vi "Prompt for Step New.vi"(8 "error in (no error)":errorcluster, 9 "Index":i32=-1, 11 "Steps":refnum<class "Step.lvclass">[](array[class])) -> (0 "error out":errorcluster, 1 "OK?":bool, 3 "Step":refnum<class "Step.lvclass">)   [LabVIEW 2020, in "MacroAssert.lvlib"]
doc: "Prompts to enter a new step in the profile."
uses:
  MacroAssert.lvlib
  Classes/Step/Step.lvclass
  CTLs/Step Type V3.ctl
  CTLs/Assertion Type.ctl
  CTLs/Prompt for Step State Data.ctl
  FaKI State Machine/FaKI State Machine.lvlib
  CTLs/Prompt for Step Front Panel Data.ctl
  <vilib>/Utility/inputDevices.llb/mouseAcquire.vi
  <vilib>/Utility/inputDevices.llb/closeMouse.vi
  <vilib>/picture/picture.llb/imagedata.ctl
  Classes/Macro/Macro.lvclass
  CTLs/Step V3.ctl
panel:
  in  "Save Default":bool
  in  "Step Notes":string
  out "Step Type Description":string
  in  "Repeat Amount":i32 min=0
  in  "Tab Control":T1(tab)
  in  "Y":i32 min=0
  in  "X":i32 min=0
  in  "Right Click?":bool
  in  "Key":u8(ring)=65
  in  "App/Window Name":string
  in  "Stop on Fail?":bool
  in  "Control Name":string
  in  "Tab Control 2":T2(tab)
  in  "Disabled":T3(ring)
  in  "Visible":enum16{"Visible", "Not Visible"}(ring)
  in  "Left":i16
  in  "Top":i16
  in  "Width":i16
  in  "Height":i16
  out "Expected Image":picture
  in  "Delay (ms)":i32=100 min=0
  in  "Step Type":T4
  in  "Cancel":bool
  in  "OK":bool caption="OK2"
  # "Left and right click at\nsame time to capture\ncurrent screen coords"
  # "Left and right click at\nsame time to capture\nexpected value"
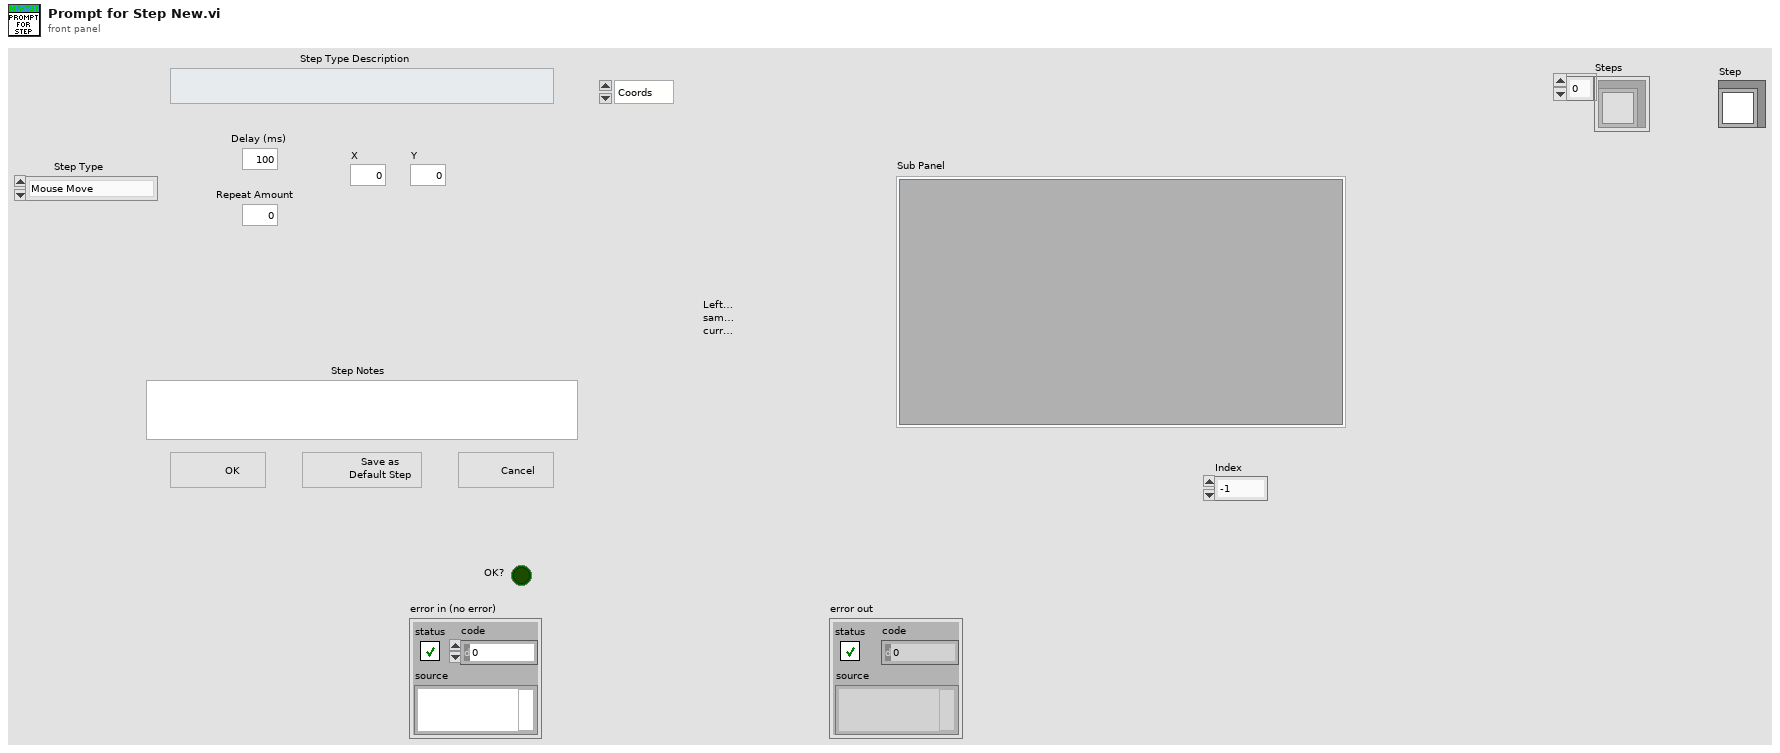
[diagram p1: front panel]
types:
  T1 = enum32{"Coords", "RClick", "Key", "A/W", "Nothing", "Assertion"}
  T2 = enum32{"Control Position", "Control Disabled", "Control Visible", "Control Image"}
  T3 = enum8{"Enabled", "Disabled", "Disabled and Grayed Out"}
  T4 = typedef "MacroAssert.lvlib/Step Type V3.ctl" = enum16{"Mouse Move", "Mouse Click", "Key Press", "Wait", "Mouse Down", "Mouse Up", "Key Down", "Key Up", "Maximize Window", "Restore Window", "Minimize Window", "Close Window", "Bring Window to Front", "Send Window to Back", "Assertion: Ctl Visible", "Assertion: Ctl Disabled", "Assertion: Ctl Image"}
  T5 = typedef "MacroAssert.lvlib/Prompt for Step State Data.ctl" = cluster{"Core":cluster{"Current VI Reference":refnum<vi>, "Close Panel on Exit?":bool}, "Mouse Ref":refnum<k1>, "Step":refnum<class "Step.lvclass">, "FP":T6, "OK?":bool}
  T6 = typedef "MacroAssert.lvlib/Prompt for Step Front Panel Data.ctl" = cluster{"Assertion Type":T7, "Step":T8}
  T7 = typedef "MacroAssert.lvlib/Assertion Type.ctl" = enum16{"Control Position", "Control Visible", "Control Disabled", "Control Image"}
  T8 = typedef "MacroAssert.lvlib/Step V3.ctl" = cluster{"Type":T4, "X":i32, "Y":i32, "Delay":i32, "Key":u8, "Repeat":i32, "RClick?":bool, "App/Window Name":string, "Notes":string, "Assertion Type":T7, "Control Name":string, "Stop on Fail?":bool, "Disabled":enum8{"Enabled", "Disabled", "Disabled and Grayed Out"}, "Visible":enum16{"Visible", "Not Visible"}, "Left":i16, "Top":i16, "Width":i16, "Height":i16, "Expected Image":T9}
  T9 = typedef "imagedata.ctl" = cluster{"image type":i32, "image depth":i32, "image":u8[], "mask":u8[], "colors":u32[], "Rectangle":cluster{"left":i16, "top":i16, "right":i16, "bottom":i16}}
  T10 = enum32{"Invalid", "Standard", "Closed", "Hidden", "Minimized", "Maximized"}
  T11 = enum32{"invalid app kind", "Development System", "Run Time System", "Student Edition", "Embedded LabVIEW", "Evaluation", "Custom"}
  T12 = enum32{"Coords", "RClick", "Key", "A/W", "Nothing"}
  T13 = cluster{"Horizontal":i32, "Vertical":i32, "Scrolling":i32}
  T14 = cluster{"button 1":bool, "button 2":bool, "button 3":bool, "button 4":bool}
  T15 = cluster{"left":i16, "top":i16, "right":i16, "bottom":i16}
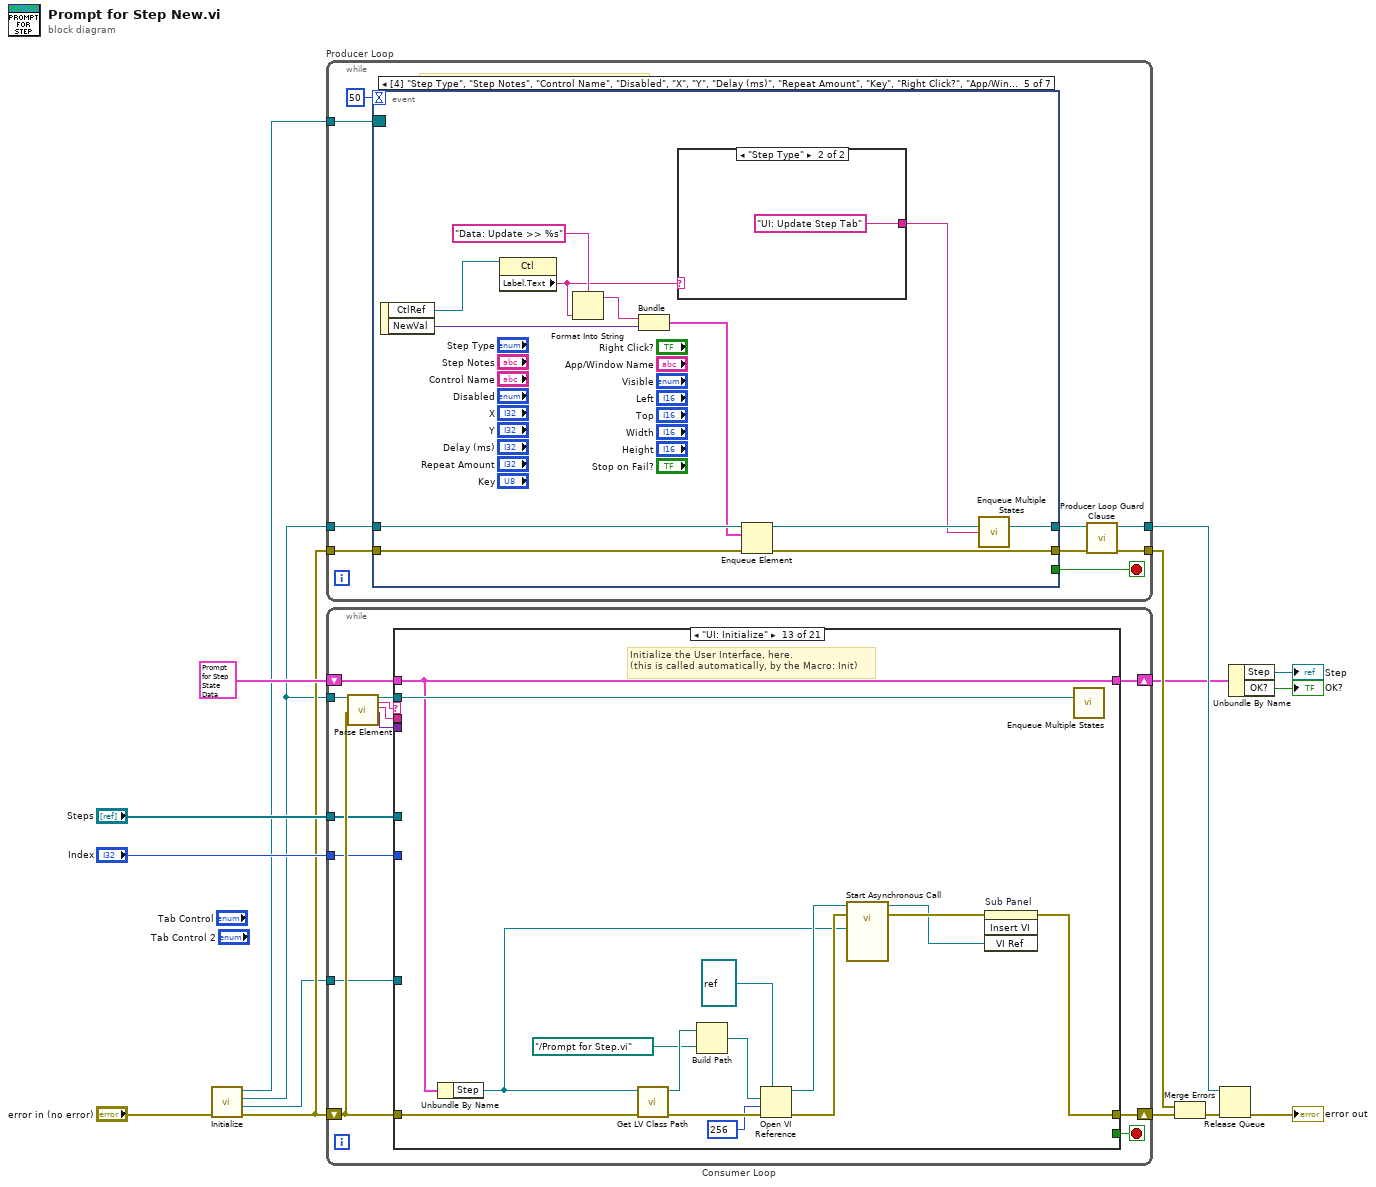
[diagram p0: block diagram]
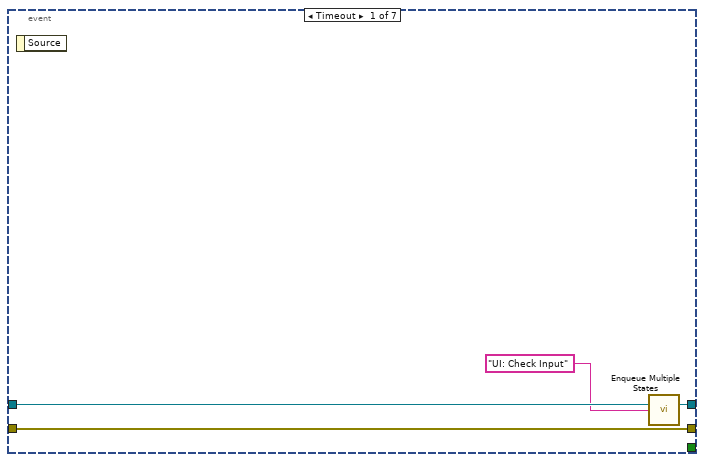
[diagram p2: hidden frame]
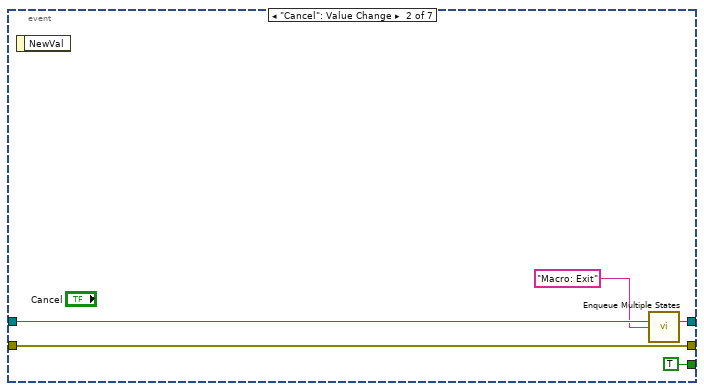
[diagram p3: hidden frame]
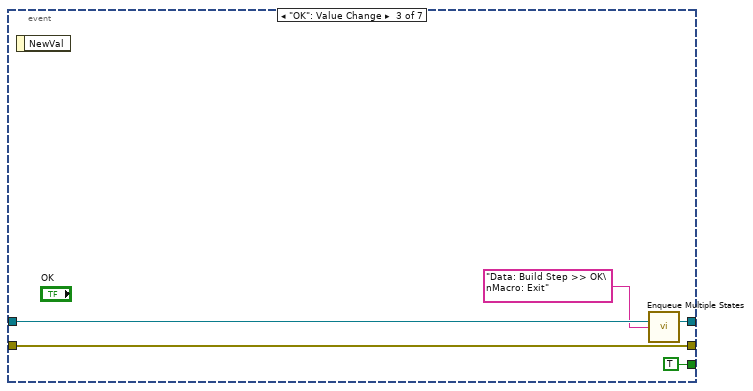
[diagram p4: hidden frame]
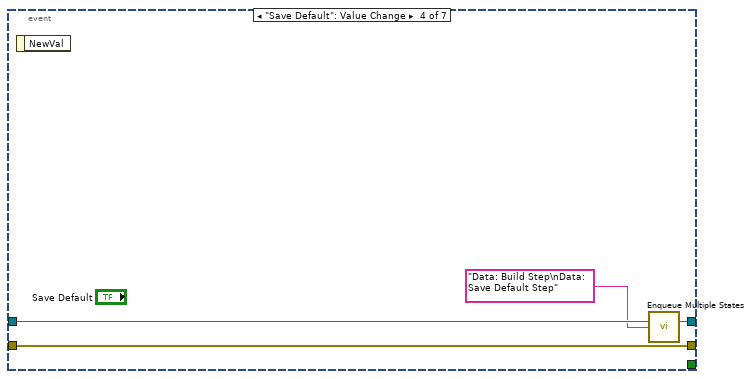
[diagram p5: hidden frame]
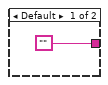
[diagram p6: hidden frame]
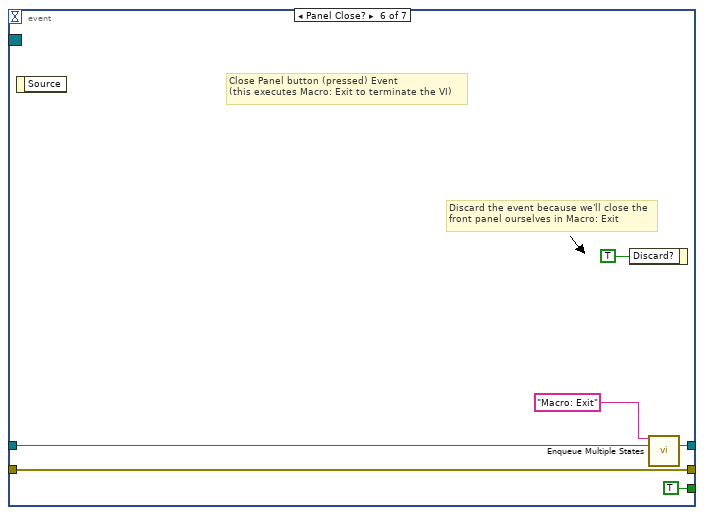
[diagram p7: hidden frame]
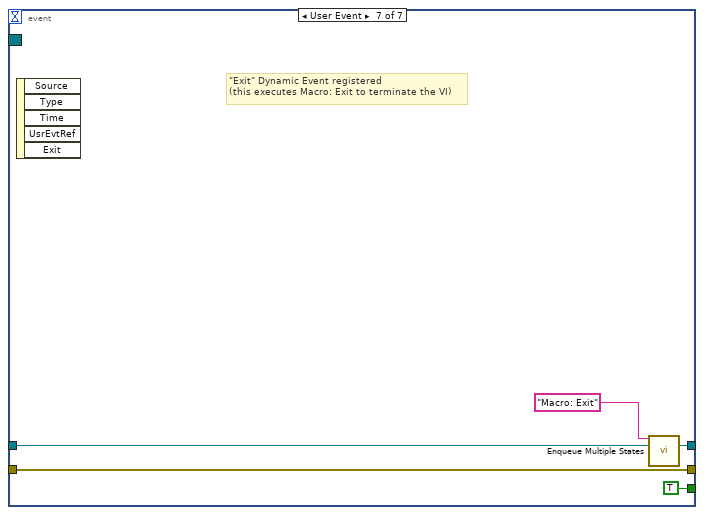
[diagram p8: hidden frame]
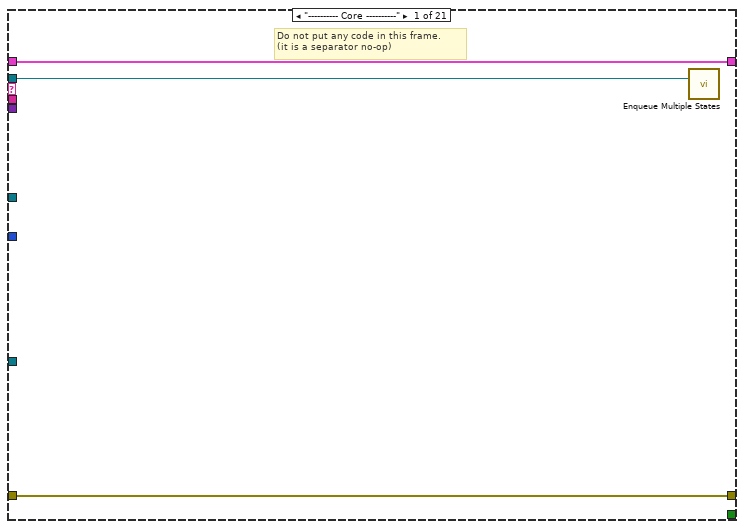
[diagram p9: hidden frame]
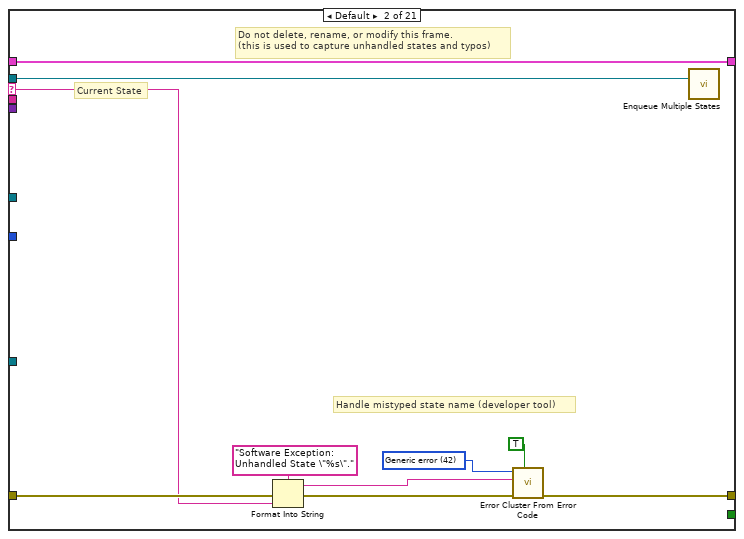
[diagram p10: hidden frame]
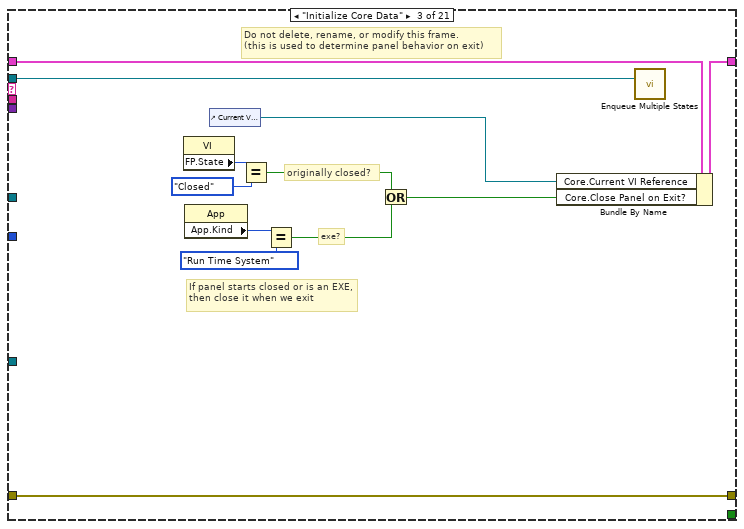
[diagram p11: hidden frame]
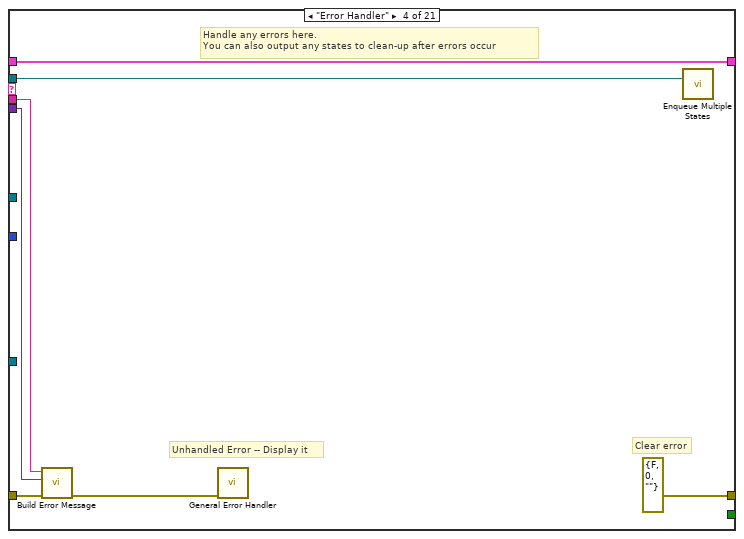
[diagram p12: hidden frame]
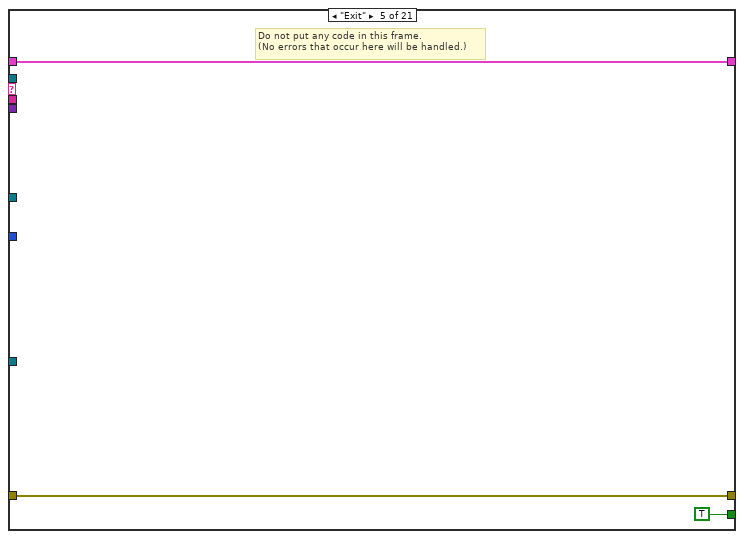
[diagram p13: hidden frame]
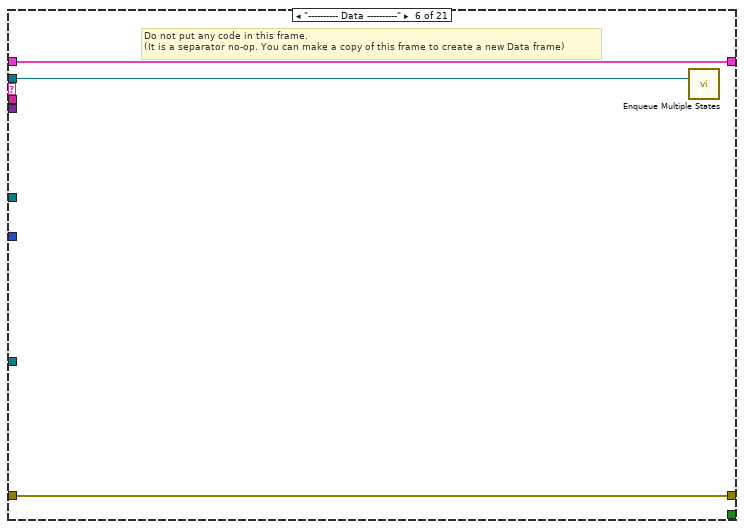
[diagram p14: hidden frame]
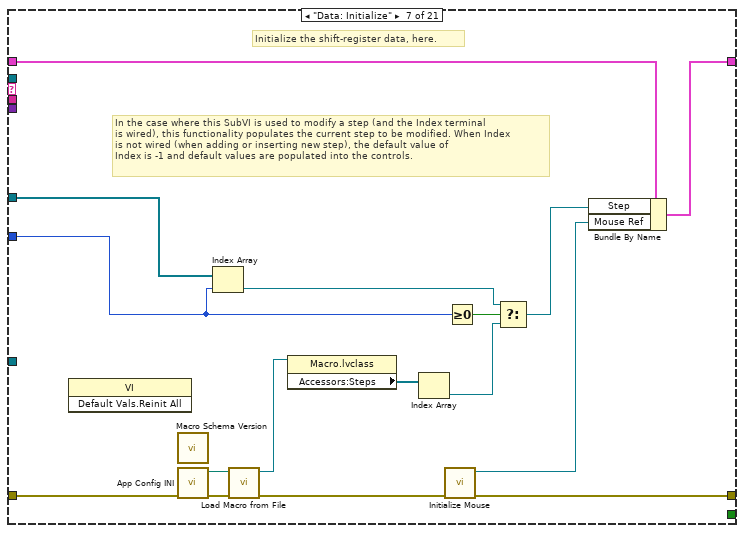
[diagram p15: hidden frame]
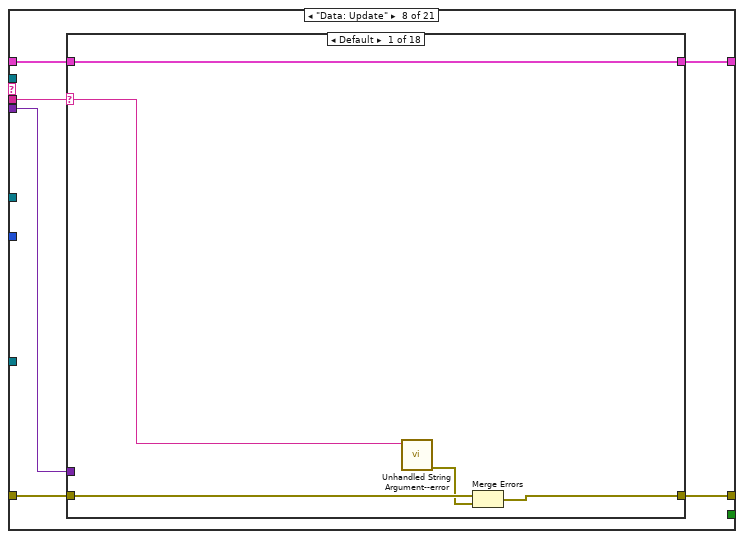
[diagram p16: hidden frame]
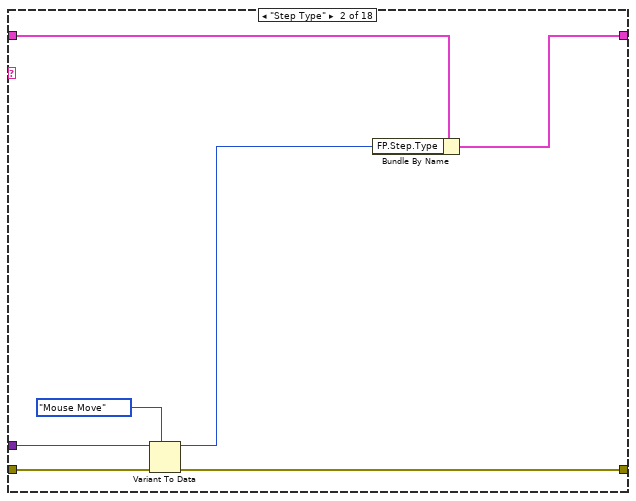
[diagram p17: hidden frame]
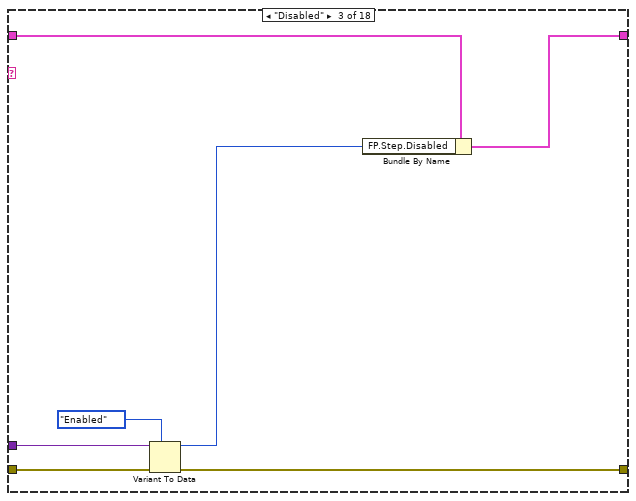
[diagram p18: hidden frame]
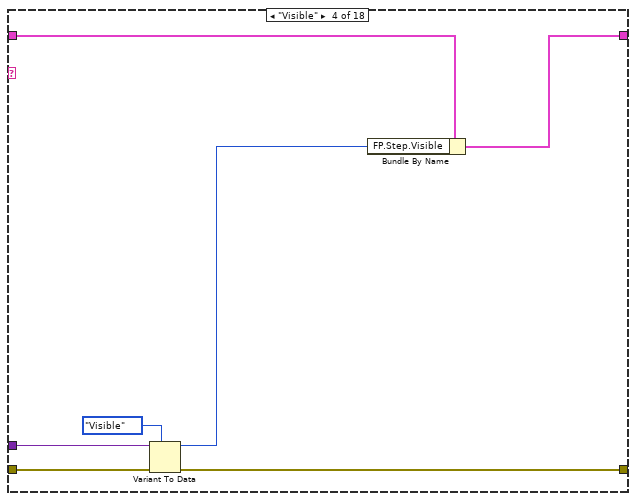
[diagram p19: hidden frame]
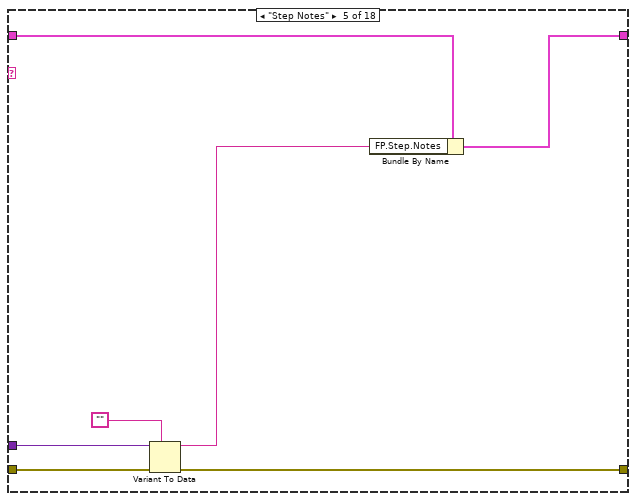
[diagram p20: hidden frame]
diagram:
  n1 = call "Initialize.vi"("error in (no error)"="error in (no error)") -> ("error out"=w5:errorcluster, "Exit Event"=w4:refnum<user-event>, "Queue"=w3:refnum<queue>, "Event Registration Refnum"=w2:refnum<event-registration>)  [unwired: 7 in]
  n2 = while "Producer Loop" {
    tunnel: w2 -> [w17]
    tunnel: w3 -> [w21]
    tunnel: [w18] -> w12
    tunnel: w5 -> [w25]
    tunnel: [w23] -> w15
    stop <- w20 stop-if-true
    # "executes when the state queue is empty"
    n3 = event shown="[4] \"Step Type\", \"Step Notes\", \"Control Name\", \"Disabled\", \"X\", \"Y\", \"Delay (ms)\", \"Repeat Amount\", \"Key\", \"Right Click?\", \"App/Window Name\", \"Visible\", \"Left\", \"Top\", \"Width\", \"Height\", \"Stop on Fail?\": Value Change" {
      selector: w17 -> [_ _ _ _ _ _ _]
      dyn-events: _ -> [_ _ _ _ _ _ _]
      timeout: 50 ("Timeout") -> [_ _ _ _ _ _ _]
      tunnel: [w29 w34 w39 w43 w54 w63 w68] -> w24
      tunnel: w25 -> [w29 w34 w39 w43 w55 w63 w68]
      tunnel: w21 -> [w27 w33 w38 w42 w53 w60 w66]
      tunnel: [w28 w32 w37 w41 w44 w59 w65] -> w19
      tunnel: [_ TRUE TRUE _ _ TRUE TRUE] -> w20
      event Timeout {
        n4 = event-data() -> ()  [unwired: 1 in, 1 out]
        n5 = call "Enqueue Multiple States.vi"("queue in"=w27, "State(s) at Back"="UI: Check Input") -> ("queue out"=w28:refnum<queue>)  [unwired: 13 in]
      }
      event "Cancel": Value Change {
        n6 = event-data() -> ()  [unwired: 1 in, 1 out]
        n7 = call "Enqueue Multiple States.vi"("queue in"=w33, "State(s) at Back"="Macro: Exit") -> ("queue out"=w32:refnum<queue>)  [unwired: 13 in]
      }
      event "OK": Value Change {
        n8 = event-data() -> ()  [unwired: 1 in, 1 out]
        n9 = call "Enqueue Multiple States.vi"("queue in"=w38, "State(s) at Back"="Data: Build Step >> OK\nMacro: Exit") -> ("queue out"=w37:refnum<queue>)  [unwired: 13 in]
      }
      event "Save Default": Value Change {
        n10 = event-data() -> ()  [unwired: 1 in, 1 out]
        n11 = call "Enqueue Multiple States.vi"("queue in"=w42, "State(s) at Back"="Data: Build Step\nData: Save Default Step") -> ("queue out"=w41:refnum<queue>)  [unwired: 13 in]
      }
      event "Step Notes", "Control Name", "Disabled", "X", "Y", "Delay (ms)", "Repeat Amount", "Key", "Right Click?", "App/Window Name", "Visible", "Left", "Top", "Width", "Height", "Stop on Fail?": Value Change {
        n12 = event-data() -> ("CtlRef"=w45:refnum<vi>, "NewVal"=w46:variant)  [unwired: 1 in]
        n13 = property class="Ctl"(reference=w45) -> ("Label.Text"=w48:string)  [unwired: 1 in, 2 out]
        n14 = Format Into String(format string="Data: Update >> %s", w48) -> (resulting string=w49:string)  [unwired: 2 in, 1 out]
        n15 = Bundle(w49, "NewVal"=w46) -> (w47:cluster{string, "NewVal":variant})  [unwired: 1 in]
        n16 = case shown="\"Step Type\"" w48 {
          tunnel: ["" ("string") "UI: Update Step Tab" ("string")] -> w51
          frame Default {
          }
          frame "Step Type" {
          }
        }
        n17 = Enqueue Element(queue=w53, element=w47, error in (no error)=w55) -> (queue out=w52:refnum<queue>, error out=w54:errorcluster)  [unwired: 1 in, 1 out]
        n18 = call "Enqueue Multiple States.vi"("queue in"=w52, "State(s) at Back"=w51) -> ("queue out"=w44:refnum<queue>)  [unwired: 13 in]
      }
      event Panel Close? {
        # "Discard the event because we'll close the front panel ourselves in Macro: Exit"
        # "Close Panel button (pressed) Event\n(this executes Macro: Exit to terminate the VI)"
        n19 = event-data() -> ()  [unwired: 1 in, 1 out]
        n20 = event-data("Discard?"=TRUE) -> ()  [unwired: 1 in, 1 out]
        n21 = call "Enqueue Multiple States.vi"("State(s) at Front"="Macro: Exit", "queue in"=w60) -> ("queue out"=w59:refnum<queue>)  [unwired: 13 in]
      }
      event User Event {
        # "\"Exit\" Dynamic Event registered\n(this executes Macro: Exit to terminate the VI)"
        n22 = event-data() -> ()  [unwired: 1 in, 5 out]
        n23 = call "Enqueue Multiple States.vi"("State(s) at Front"="Macro: Exit", "queue in"=w66) -> ("queue out"=w65:refnum<queue>)  [unwired: 13 in]
      }
    }
    n24 = call "Producer Loop Guard Clause.vi"("error in (no error)"=w24, "queue in"=w19) -> ("error out"=w23:errorcluster, "queue out"=w18:refnum<queue>)  [unwired: 8 in]
  }
  n25 = while "Consumer Loop" {
    shift-right: [w78] -> w8
    shift-left: T5 {"Core"={"Current VI Reference"=refnum, "Close Panel on Exit?"=FALSE}, "Mouse Ref"=refnum, "Step"=refnum, "FP"={"Assertion Type"=enum."Control Position", "Step"={"Type"=enum."Mouse Move", "X"=0, "Y"=0, "Delay"=0, "Key"=0, "Repeat"=0, "RClick?"=FALSE, "App/Window Name"="", "Notes"="", "Assertion Type"=enum."Control Position", "Control Name"="", "Stop on Fail?"=FALSE, "Disabled"=enum."Enabled", "Visible"=enum."Visible", "Left"=0, "Top"=0, "Width"=0, "Height"=0, "Expected Image"={"image type"=0, "image depth"=0, "image"=[], "mask"=[], "colors"=[], "Rectangle"={"left"=0, "top"=0, "right"=0, "bottom"=0}}}}, "OK?"=FALSE} ("Prompt for Step State Data") -> [w69]
    shift-right: [w81] -> w16
    shift-left: w5 -> [w80]
    tunnel: w3 -> [w77]
    tunnel: w4 -> [w72]
    tunnel: "Steps" -> [w71]
    tunnel: "Index" -> [w70]
    stop <- w79 stop-if-true
    n26 = call "Parse Element.vi"("queue in"=w77, "error in (no error)"=w80) -> ("queue out"=w76:refnum<queue>, "State"=w75:string, "Arg"=w74:string, "Data"=w73:variant)  [unwired: 14 in]
    n27 = case shown="\"UI: Initialize\"" w75 {
      selector: w75 -> [_ w86 _ _ _ _ _ _ _ _ _ _ _ _ _ _ _ _ _ _ _]
      tunnel: w76 -> [w82 w85 w95 w109 _ w117 _ _ _ _ w291 w297 w314 w317 w318 w327 _ _ w496 w501 w507]
      tunnel: w74 -> [_ _ _ w107 _ _ _ w138 _ w285 _ _ _ _ w319 w328 _ _ _ _ _]
      tunnel: w69 -> [w83 w88 w101 w110 w115 w118 w133 w139 w275 w287 w292 w298 w308 w316 w320 w330 w400 w443 w497 w500 w511]
      tunnel: [w84 w93 w106 errorcluster {"status"=FALSE, "code"=0, "source"=""} ("error out") w116 w119 w134 w140 w268 w279 w294 w299 w300 w315 w321 w331 w403 w445 w498 w502 w512] -> w81
      tunnel: w80 -> [w84 w92 w106 w112 w116 w119 w135 w141 w276 w282 w296 w299 w309 w315 w322 w332 w403 w446 w498 w502 w512]
      tunnel: [_ _ _ _ TRUE _ _ _ _ _ _ _ _ _ _ _ _ _ _ _ _] -> w79
      tunnel: [w83 w88 w105 w110 w115 w118 w132 w136 w275 w286 w292 w298 w308 w316 w320 w330 w400 w442 w497 w500 w511] -> w78
      tunnel: w73 -> [_ _ _ w108 _ _ _ w137 _ _ _ _ _ _ _ _ _ _ _ _ _]
      tunnel: w72 -> [_ _ _ _ _ _ _ _ _ _ _ _ _ _ _ _ _ _ _ _ _]
      tunnel: w71 -> [_ _ _ _ _ _ w129 _ _ _ _ _ _ _ _ _ _ _ _ _ _]
      tunnel: w70 -> [_ _ _ _ _ _ w128 _ _ _ _ _ _ _ _ _ _ _ _ _ _]
      frame "---------- Core ----------" {
        # "Do not put any code in this frame.\n(it is a separator no-op)"
        n28 = call "Enqueue Multiple States.vi"("queue in"=w82) -> ()  [unwired: 14 in, 1 out]
      }
      frame Default {
        w90 = 42 items=["No error", "Argument error", "Memory is full", "Out of zone", "End of file", "File already open", "Generic file I/O error", "File not found", "File permission error", "Disk is full", "Duplicate path", "Too many files open", "System feature not enabled", "Resource file not found", "Cannot add resource", "Resource not found", "Image not found", "Image memory error", "Pen does not exist", "Config type invalid", "Config token not found", "Config parse error", "Config memory error", "Bad external code format", "Bad external code offset", "External code not present", "Null window", "Destroy window error", "Null menu", "Print aborted", "Bad print record", "Print driver error", "Windows error during printing", "Memory error during printing", "Print dialog error", "Generic print error", "Invalid device refnum", "Device not found", "Device parameter error", "Device unit error", "Cannot open device", "Device call aborted", "Generic error", "Cancelled by user", "Object ID too low", "Object ID too high", "Object not in heap", "Unknown heap", "Unknown object (invalid DefProc)", "Unknown object (DefProc not in table)", "Message out of range", "Invalid (null) method", "Unknown message", "Manager call not supported", "Bad address", "Network operation in progress", "Network operation timed out", "Connection is busy", "Network attribute not supported", "Network error", "Address in use", "System out of memory", "Connection aborted", "Connection refused", "Not connected", "Already connected", "Connection closed", "Initialization error (interapplication manager)", "Bad occurrence", "Wait on unbound occurrence handler", "Occurrence queue overflow", "Datalog type conflict", "Unused", "Unrecognized type (interapplication manager)", "Memory corrupt", "Failed to make temporary DLL", "Old CIN version", "Drag socket not found", "Failed to load drop-object", "Failed to register OLE object", "Failed to release OLE object", "Format specifier type mismatch", "Unknown format specifier", "Too few format specifiers", "Too many format specifiers", "Scan failed", "Newer CIN version", "Error converting to variant", "Runtime menu error", "Password tampered", "Variant attribute not found", "Incompatible variant data type", "Event data is not available", "Event Store is not present", "Occurrence is not found", "Event Queue is not created", "Event info is not available", "Refnum passed is NULL", "Error retrieving Class GUID", "Error retrieving CoClass GUID", "Error retrieving TypeLib GUID.", "Bad built application magic bytes.", "Specific driver is different from the specific driver associated with the Logical Name.", "There is no session opened to the class driver.", "Max Error", "MAX - Error with config objects", "MAX - Error loading configuration", "MAX - Group not supported"]
        # "Current State"
        # "Do not delete, rename, or modify this frame.\n(this is used to capture unhandled states and typos)"
        # "Handle mistyped state name (developer tool)"
        n29 = Format Into String(format string="Software Exception: Unhandled State \"%s\"." ("message"), error in=w92, w86) -> (resulting string=w89:string, error out=w94:errorcluster)  [unwired: 1 in]
        n30 = call <vilib>:"Error Cluster From Error Code.vi"("show call chain? (False)"=TRUE, "error in (no error)"=w94, "error message (\"\")"=w89, "error code (0)"=w90) -> ("error out"=w93:errorcluster)  [unwired: 5 in]
        n31 = call "Enqueue Multiple States.vi"("queue in"=w85) -> ()  [unwired: 14 in, 1 out]
      }
      frame "Initialize Core Data" {
        # "Do not delete, rename, or modify this frame.\n(this is used to determine panel behavior on exit)"
        # "originally closed?"
        # "exe?"
        # "If panel starts closed or is an EXE, then close it when we exit"
        n32 = property class="VI"() -> ("FP.State"=w98:T10)  [unwired: 2 in, 2 out]
        n33 = property class="App"() -> ("App.Kind"=w104:T11)  [unwired: 2 in, 2 out]
        n34 = control-ref of="Current VI Reference"() -> (w99:refnum<vi>)
        n35 = Equal?(x=w98, y=T10."Closed" ("Front Panel Window:State")) -> (x = y?=w96:bool)
        n36 = Equal?(x=w104, y=T11."Run Time System" ("Application:Kind")) -> (x = y?=w102:bool)
        n37 = Or(x=w96, y=w102) -> (x .or. y?=w100:bool)
        n38 = Bundle By Name(cluster=w101, "Core.Current VI Reference"=w99, "Core.Close Panel on Exit?"=w100) -> (w105:T5)
        n39 = call "Enqueue Multiple States.vi"("queue in"=w95) -> ()  [unwired: 14 in, 1 out]
      }
      frame "Error Handler" {
        # "Unhandled Error -- Display it"
        # "Handle any errors here.\nYou can also output any states to clean-up after errors occur"
        # "Clear error"
        n40 = call "Build Error Message.vi"("error in (no error)"=w112, "Data"=w108, "Arg"=w107) -> ("error out"=w111:errorcluster)  [unwired: 8 in]
        n41 = call <vilib>:"General Error Handler.vi"("error in (no error)"=w111) -> ()  [unwired: 10 in, 5 out]
        n42 = call "Enqueue Multiple States.vi"("queue in"=w109) -> ()  [unwired: 14 in, 1 out]
      }
      frame "Exit" {
        # "Do not put any code in this frame.\n(No errors that occur here will be handled.)"
      }
      frame "---------- Data ----------" {
        # "Do not put any code in this frame.\n(It is a separator no-op. You can make a copy of this frame to create a new Data frame)"
        n43 = call "Enqueue Multiple States.vi"("queue in"=w117) -> ()  [unwired: 14 in, 1 out]
      }
      frame "Data: Initialize" {
        # "In the case where this SubVI is used to modify a step (and the Index terminal\nis wired), this functionality populates the current step to be modified. When Index\nis not wired (when adding or inserting new step), the default value of\nIndex is -1 and default values are populated into the controls."
        # "Initialize the shift-register data, here."
        n44 = invoke class="VI" method="Default Vals.Reinit All"() -> ()  [unwired: 3 in, 3 out]
        n45 = call "Macro Schema Version.vi"() -> ()  [unwired: 10 in, 2 out]
        n46 = call "App Config INI.vi"("error in (no error)"=w135) -> ("error out"=w125:errorcluster, "App Config"=w124:path)  [unwired: 9 in]
        n47 = Index Array(array=w129, index=w128) -> (element=w131:refnum<class "Step.lvclass">)
        n48 = call "Load Macro from File.vi"("error in (no error)"=w125, "Path"=w124) -> ("error out"=w123:errorcluster, "Macro"=w121:refnum<class "Macro.lvclass">)  [unwired: 8 in]
        n49 = property class="Macro.lvclass"(reference=w121) -> ("Accessors:Steps"=w120:refnum<class "Step.lvclass">[])  [unwired: 1 in, 2 out]
        n50 = Index Array(array=w120) -> (element=w122:refnum<class "Step.lvclass">)  [unwired: 1 in]
        n51 = call <vilib>:"Initialize Mouse.vi"("error in (no error)"=w123) -> ("error out"=w134:errorcluster, "device ID"=w126:refnum<k1>)  [unwired: 9 in]
        n52 = Greater Or Equal To 0?(x=w128) -> (x >= 0?=w130:bool)
        n53 = Select(t=w131, s=w130, f=w122) -> (s? t:f=w127:refnum<class "Step.lvclass">)
        n54 = Bundle By Name(cluster=w133, "Step"=w127, "Mouse Ref"=w126) -> (w132:T5)
      }
      frame "Data: Update" {
        n55 = case shown="Default" w138 {
          selector: w138 -> [w142 _ _ _ _ _ _ _ _ _ _ _ _ _ _ _ _ _]
          tunnel: w141 -> [w146 w153 w160 w167 w174 w181 w188 w195 w202 w209 w216 w223 w230 w237 w244 w251 w258 w265]
          tunnel: w139 -> [w144 w149 w157 w164 w171 w178 w185 w192 w199 w206 w213 w220 w227 w234 w241 w248 w255 w262]
          tunnel: w137 -> [_ w150 w158 w165 w172 w179 w186 w193 w200 w207 w214 w221 w228 w235 w242 w249 w256 w263]
          tunnel: [w144 w148 w156 w163 w170 w177 w184 w191 w198 w205 w212 w219 w226 w233 w240 w247 w254 w261] -> w136
          tunnel: [w145 w152 w159 w166 w173 w180 w187 w194 w201 w208 w215 w222 w229 w236 w243 w250 w257 w264] -> w140
          frame Default {
            n56 = call "Unhandled String Argument--error.vi"("Control Name"=w142) -> ("error out"=w143:errorcluster)  [unwired: 10 in]
            n57 = Merge Errors(w146, w143) -> (w145:errorcluster)
          }
          frame "Step Type" {
            n58 = Variant To Data(error in=w153, type=Step_Type_V3."Mouse Move" ("Type"), Variant=w150) -> (data=w147:T4, error out=w152:errorcluster)
            n59 = Bundle By Name(cluster=w149, "FP.Step.Type"=w147) -> (w148:T5)
          }
          frame "Disabled" {
            n60 = Variant To Data(error in=w160, type=T3."Enabled" ("Disabled"), Variant=w158) -> (data=w155:T3, error out=w159:errorcluster)
            n61 = Bundle By Name(cluster=w157, "FP.Step.Disabled"=w155) -> (w156:T5)
          }
          frame "Visible" {
            n62 = Variant To Data(error in=w167, type=enum16{"Visible", "Not Visible"}."Visible" ("Visible"), Variant=w165) -> (data=w162:enum16{"Visible", "Not Visible"}, error out=w166:errorcluster)
            n63 = Bundle By Name(cluster=w164, "FP.Step.Visible"=w162) -> (w163:T5)
          }
          frame "Step Notes" {
            n64 = Variant To Data(error in=w174, type="", Variant=w172) -> (data=w169:string, error out=w173:errorcluster)
            n65 = Bundle By Name(cluster=w171, "FP.Step.Notes"=w169) -> (w170:T5)
          }
          frame "App/Window Name" {
            n66 = Variant To Data(error in=w181, type="", Variant=w179) -> (data=w176:string, error out=w180:errorcluster)
            n67 = Bundle By Name(cluster=w178, "FP.Step.App/Window Name"=w176) -> (w177:T5)
          }
          frame "Control Name" {
            n68 = Variant To Data(error in=w188, type="", Variant=w186) -> (data=w183:string, error out=w187:errorcluster)
            n69 = Bundle By Name(cluster=w185, "FP.Step.Control Name"=w183) -> (w184:T5)
          }
          frame "X" {
            n70 = Variant To Data(error in=w195, type=0, Variant=w193) -> (data=w190:i32, error out=w194:errorcluster)
            n71 = Bundle By Name(cluster=w192, "FP.Step.X"=w190) -> (w191:T5)
          }
          frame "Y" {
            n72 = Variant To Data(error in=w202, type=0, Variant=w200) -> (data=w197:i32, error out=w201:errorcluster)
            n73 = Bundle By Name(cluster=w199, "FP.Step.Y"=w197) -> (w198:T5)
          }
          frame "Delay (ms)" {
            n74 = Variant To Data(error in=w209, type=0, Variant=w207) -> (data=w204:i32, error out=w208:errorcluster)
            n75 = Bundle By Name(cluster=w206, "FP.Step.Delay"=w204) -> (w205:T5)
          }
          frame "Repeat Amount" {
            n76 = Variant To Data(error in=w216, type=0, Variant=w214) -> (data=w211:i32, error out=w215:errorcluster)
            n77 = Bundle By Name(cluster=w213, "FP.Step.Repeat"=w211) -> (w212:T5)
          }
          frame "Left" {
            n78 = Variant To Data(error in=w223, type=i16 0, Variant=w221) -> (data=w218:i16, error out=w222:errorcluster)
            n79 = Bundle By Name(cluster=w220, "FP.Step.Left"=w218) -> (w219:T5)
          }
          frame "Top" {
            n80 = Variant To Data(error in=w230, type=i16 0, Variant=w228) -> (data=w225:i16, error out=w229:errorcluster)
            n81 = Bundle By Name(cluster=w227, "FP.Step.Top"=w225) -> (w226:T5)
          }
          frame "Width" {
            n82 = Variant To Data(error in=w237, type=i16 0, Variant=w235) -> (data=w232:i16, error out=w236:errorcluster)
            n83 = Bundle By Name(cluster=w234, "FP.Step.Width"=w232) -> (w233:T5)
          }
          frame "Height" {
            n84 = Variant To Data(error in=w244, type=i16 0, Variant=w242) -> (data=w239:i16, error out=w243:errorcluster)
            n85 = Bundle By Name(cluster=w241, "FP.Step.Height"=w239) -> (w240:T5)
          }
          frame "Key" {
            n86 = Variant To Data(error in=w251, type=u8 65 ("Key"), Variant=w249) -> (data=w246:u8, error out=w250:errorcluster)
            n87 = Bundle By Name(cluster=w248, "FP.Step.Key"=w246) -> (w247:T5)
          }
          frame "Right Click?" {
            n88 = Variant To Data(error in=w258, type=FALSE, Variant=w256) -> (data=w253:bool, error out=w257:errorcluster)
            n89 = Bundle By Name(cluster=w255, "FP.Step.RClick?"=w253) -> (w254:T5)
          }
          frame "Stop on Fail?" {
            n90 = Variant To Data(error in=w265, type=FALSE, Variant=w263) -> (data=w260:bool, error out=w264:errorcluster)
            n91 = Bundle By Name(cluster=w262, "FP.Step.Stop on Fail?"=w260) -> (w261:T5)
          }
        }
      }
      frame "Data: Save Default Step" {
        n92 = Unbundle By Name(w275) -> ("Step"=w274:refnum<class "Step.lvclass">)
        n93 = Build Array(w274) -> (w266:refnum<class "Step.lvclass">[])
        n94 = call "App Config INI.vi"("error in (no error)"=w276) -> ("error out"=w273:errorcluster, "App Config"=w272:path)  [unwired: 9 in]
        n95 = call-dynamic "Initialize.vi"("error in (no error)"=w273, "Path"=w272, "Macro in"=refnum<class "Macro.lvclass"> refnum) -> ("error out"=w270:errorcluster, "Macro out"=w269:refnum<class "Macro.lvclass">)  [unwired: 7 in]
        n96 = property class="Macro.lvclass"(reference=w269, "Accessors:Steps"=w266) -> (reference out=w267:refnum<class "Macro.lvclass">)  [unwired: 1 in, 1 out]
        n97 = call-dynamic "Write to File.vi"("error in (no error)"=w270, "Macro in"=w267) -> ("error out"=w268:errorcluster)  [unwired: 8 in, 1 out]
      }
      frame "Data: Build Step" {
        n98 = Equal?(x=w285, y="OK") -> (x = y?=w278:bool)
        n99 = Unbundle By Name(w287) -> ("FP.Step"=w288:T8, "FP.Step.Type"=w277:T4)
        n100 = call "Load Step.vi"("error in (no error)"=w282, "Index"=0, "Step Type"=w277) -> ("error out"=w280:errorcluster, "Step"=w289:refnum<class "Step.lvclass">)  [unwired: 7 in]
        n101 = call-dynamic "Set All Parameters.vi"("error in (no error)"=w280, "Parameters"=w288, "Step in"=w289) -> ("error out"=w279:errorcluster, "Step out"=w281:refnum<class "Step.lvclass">)  [unwired: 7 in]
        n102 = Bundle By Name(cluster=w287, "Step"=w281, "OK?"=w278) -> (w286:T5)
      }
      frame "Data: Cleanup" {
        # "Cleanup any data and references, here.\n(this is called automatically, by the Macro: Exit)"
        n103 = Unbundle By Name(w292) -> ("Mouse Ref"=w290:refnum<k1>, "Core.Current VI Reference"=w293:refnum<vi>)
        n104 = Close Reference(reference=w293, error in (no error)=w296) -> (error out=w295:errorcluster)
        n105 = call-poly <vilib>:"Close Input Device.vi"("error in (no error)"=w295, "device ID"=w290) -> ("error out"=w294:errorcluster)  [unwired: 8 in]
        n106 = call "Enqueue Multiple States.vi"("queue in"=w291) -> ()  [unwired: 14 in, 1 out]
      }
      frame "---------- UI ----------" {
        # "Do not put any code in this frame.\n(It is a separator no-op. You can make a copy of this frame to create a new UI frame)"
        n107 = call "Enqueue Multiple States.vi"("queue in"=w297) -> ()  [unwired: 14 in, 1 out]
      }
      frame "UI: Initialize" {
        # "Initialize the User Interface, here.\n(this is called automatically, by the Macro: Init)"
        n108 = Unbundle By Name(w308) -> ("Step"=w303:refnum<class "Step.lvclass">)
        n109 = call <vilib>:"Get LV Class Path.vi"("error in (no error)"=w309, "object"=w303) -> ("error out"=w313:errorcluster, "class path"=w311:path)  [unwired: 8 in]
        n110 = Build Path(base path=w311, name or relative path=path "../Prompt for Step.vi") -> (appended path=w312:path)
        n111 = Open VI Reference(type specifier VI Refnum (for type only)=refnum<vi> refnum, vi path=w312, options=256, error in (no error)=w313) -> (vi reference=w306:refnum<vi>, error out=w304:errorcluster)  [unwired: 2 in]
        n112 = call-by-ref "Start Asynchronous Call"(reference=w306, error in=w304, "Step in"=w303) -> (reference out=w301:refnum<vi>, error out=w302:errorcluster)  [unwired: 8 in, 3 out]
        n113 = invoke on="Sub Panel" class="SubPnl" method="Insert VI"(error in=w302, "VI Ref"=w301) -> (error out=w300:errorcluster)  [unwired: 2 in, 3 out]
        n114 = call "Enqueue Multiple States.vi"("queue in"=w314) -> ()  [unwired: 14 in, 1 out]
      }
      frame "UI: Uninitialize" {
        # "Uninitialize the User Interface, here.\n(this is called automatically, by the Macro: Exit)"
        n115 = call "Enqueue Multiple States.vi"("queue in"=w317) -> ()  [unwired: 14 in, 1 out]
      }
      frame "UI: Cursor Set" {
        # "Argument"
        # "Set and Unset Cursor Busy.\n(Usage: \"UI: Cursor Set >> Busy|Idle\")"
        n116 = case shown="\"Idle\", Default" w319 {
          tunnel: w322 -> [w324 w326]
          tunnel: [w323 w325] -> w321
          frame "Idle", Default {
            n117 = call <vilib>:"Unset Busy.vi"("error in (no error)"=w324) -> ("error out"=w323:errorcluster)  [unwired: 10 in]
          }
          frame "Busy" {
            n118 = call <vilib>:"Set Busy.vi"("error in (no error)"=w326) -> ("error out"=w325:errorcluster)  [unwired: 9 in, 1 out]
          }
        }
        n119 = call "Enqueue Multiple States.vi"("queue in"=w318) -> ()  [unwired: 14 in, 1 out]
      }
      frame "UI: Front Panel State" {
        # "Argument"
        # "Set Front Panel Open or Closed\n(Usage: \"UI: Front Panel State >> Open|Close\")"
        n120 = Unbundle By Name(w330) -> ("Core.Current VI Reference"=w329:refnum<vi>)
        n121 = case shown="\"Open\", \"Standard\", Default" w328 {
          tunnel: w332 -> [w339 w353 w365 w378 w391]
          tunnel: [w340 w354 w366 w379 w392] -> w331
          tunnel: w329 -> [w337 w351 w363 w376 w389]
          frame "Open", "Standard", Default {
            w333 = T10."Standard" ("State")
            n122 = property class="VI"(reference=w337, error in=w339) -> (reference out=w336:refnum<vi>, error out=w338:errorcluster, "FP.State"=w335:T10)
            n123 = Not Equal?(x=w335, y=w333) -> (x != y?=w334:bool)
            n124 = case shown="True" w334 {
              tunnel: [w345 w346] -> w340
              tunnel: w338 -> [w344 w346]
              tunnel: w336 -> [w342 _]
              tunnel: w333 -> [w341 _]
              frame True {
                n125 = invoke class="VI" method="FP.Open"(reference=w342, error in=w344, "Activate"=TRUE, "State"=w341) -> (error out=w345:errorcluster)  [unwired: 1 in, 4 out]
              }
              frame False {
              }
            }
          }
          frame "Close", "Closed" {
            n126 = property class="VI"(reference=w351, error in=w353) -> (reference out=w350:refnum<vi>, error out=w352:errorcluster, "FP.State"=w348:T10)
            n127 = Not Equal?(x=w348, y=T10."Closed" ("Front Panel Window:State")) -> (x != y?=w347:bool)
            n128 = case shown="True" w347 {
              tunnel: [w355 w358] -> w354
              tunnel: w352 -> [w355 w357]
              tunnel: w350 -> [_ w356]
              frame False {
              }
              frame True {
                n129 = invoke class="VI" method="FP.Close"(reference=w356, error in=w357) -> (error out=w358:errorcluster)  [unwired: 1 in, 2 out]
              }
            }
          }
          frame "Hidden", "Hide" {
            w359 = T10."Hidden" ("State")
            n130 = property class="VI"(reference=w363, error in=w365) -> (reference out=w362:refnum<vi>, error out=w364:errorcluster, "FP.State"=w361:T10)
            n131 = Not Equal?(x=w361, y=w359) -> (x != y?=w360:bool)
            n132 = case shown="True" w360 {
              tunnel: [w370 w371] -> w366
              tunnel: w364 -> [w369 w371]
              tunnel: w362 -> [w368 _]
              tunnel: w359 -> [w367 _]
              frame True {
                n133 = invoke class="VI" method="FP.Open"(reference=w368, error in=w369, "State"=w367) -> (error out=w370:errorcluster)  [unwired: 2 in, 4 out]
              }
              frame False {
              }
            }
          }
          frame "Minimize", "Minimized" {
            w372 = T10."Minimized" ("State")
            n134 = property class="VI"(reference=w376, error in=w378) -> (reference out=w375:refnum<vi>, error out=w377:errorcluster, "FP.State"=w374:T10)
            n135 = Not Equal?(x=w374, y=w372) -> (x != y?=w373:bool)
            n136 = case shown="True" w373 {
              tunnel: [w383 w384] -> w379
              tunnel: w377 -> [w382 w384]
              tunnel: w375 -> [w381 _]
              tunnel: w372 -> [w380 _]
              frame True {
                n137 = invoke class="VI" method="FP.Open"(reference=w381, error in=w382, "State"=w380) -> (error out=w383:errorcluster)  [unwired: 2 in, 4 out]
              }
              frame False {
              }
            }
          }
          frame "Maximize", "Maximized" {
            w385 = T10."Maximized" ("State")
            n138 = property class="VI"(reference=w389, error in=w391) -> (reference out=w388:refnum<vi>, error out=w390:errorcluster, "FP.State"=w387:T10)
            n139 = Not Equal?(x=w387, y=w385) -> (x != y?=w386:bool)
            n140 = case shown="True" w386 {
              tunnel: [w396 w397] -> w392
              tunnel: w390 -> [w395 w397]
              tunnel: w388 -> [w394 _]
              tunnel: w385 -> [w393 _]
              frame True {
                n141 = invoke class="VI" method="FP.Open"(reference=w394, error in=w395, "State"=w393) -> (error out=w396:errorcluster)  [unwired: 2 in, 4 out]
              }
              frame False {
              }
            }
          }
        }
        n142 = call "Enqueue Multiple States.vi"("queue in"=w327) -> ()  [unwired: 14 in, 1 out]
      }
      frame "UI: Update Step Tab" {
        n143 = Unbundle By Name(w400) -> ("FP.Step.Type"=w399:T4)
        n144 = case shown="\"Assertion: Ctl Visible\"" w399 {
          tunnel: ["Moves mouse to desired coordinates, then waits for delay time amount" "Clicks mouse down and waits for half delay time, then clicks mouse up and waits for half delay time amount" "Presses key down and waits for half delay time, then presses key up and waits for half delay time amount" "Waits for delay time amount" "Clicks mouse down and waits for delay time amount" "Clicks mouse up and waits for delay time amount" "Presses key down and waits for delay time amount" "Presses key up and waits for delay time amount" "Tests that a control has a certain Visible value" "Tests that a control has a certain Disabled value" "Tests that a portion of a control's image is a certain value" "Maximizes a window by the given window name" "Restores (unmaximizes) a window by the given window name" "Minimizes a window by the given window name" "Closes a window by the given window name" "Puts a window in front of all other windows by the given window name" "Puts a window behind all other windows by the given window name"] -> w402
          tunnel: [T12."Coords" ("Tab Control") T12."RClick" ("Tab Control") T12."Key" ("Tab Control") T12."Nothing" ("Tab Control") T12."RClick" ("Tab Control") T12."RClick" ("Tab Control") T12."Key" ("Tab Control") T12."Key" ("Tab Control") T1."Assertion" ("Tab Control") T1."Assertion" ("Tab Control") T1."Assertion" ("Tab Control") T12."A/W" ("Tab Control") T12."A/W" ("Tab Control") T12."A/W" ("Tab Control") T12."A/W" ("Tab Control") T12."A/W" ("Tab Control") T12."A/W" ("Tab Control")] -> w401
          tunnel: [_ _ _ _ _ _ _ _ T2."Control Visible" ("Tab Control 2") T2."Control Disabled" ("Tab Control 2") T2."Control Image" ("Tab Control 2") _ _ _ _ _ _] -> w398
          frame "Mouse Move" {
          }
          frame "Mouse Click" {
          }
          frame "Key Press" {
          }
          frame "Wait" {
          }
          frame "Mouse Down" {
          }
          frame "Mouse Up" {
          }
          frame "Key Down" {
          }
          frame "Key Up" {
          }
          frame "Assertion: Ctl Visible" {
          }
          frame "Assertion: Ctl Disabled" {
          }
          frame "Assertion: Ctl Image" {
          }
          frame "Maximize Window" {
          }
          frame "Restore Window" {
          }
          frame "Minimize Window" {
          }
          frame "Close Window" {
          }
          frame "Bring Window to Front" {
          }
          frame "Send Window to Back" {
          }
        }
        "Step Type Description" <- w402
        n145 = property on="Tab Control" class="TabCtl (strict)"("Value"=w401) -> ()  [unwired: 2 in, 2 out]
        n146 = property on="Tab Control 2" class="TabCtl (strict)"("Value"=w398) -> ()  [unwired: 2 in, 2 out]
      }
      frame "UI: Check Input" {
        n147 = local read "Tab Control"() -> (w441:T1)
        n148 = Unbundle By Name(w443) -> ("Mouse Ref"=w444:refnum<k1>)
        n149 = case shown="\"Assertion\"" w441 {
          tunnel: w446 -> [w458 w479 w495]
          tunnel: w444 -> [w456 w476 _]
          tunnel: [w457 w477 w495] -> w445
          tunnel: w443 -> [w448 w470 w494]
          tunnel: [w447 w471 w494] -> w442
          frame "Coords" {
            n150 = call-poly <vilib>:"Acquire Input Data.vi"("device ID"=w456, "error in (no error)"=w458) -> ("axis info"=w454:T13, "button info"=w455:T14, "error out"=w457:errorcluster)  [unwired: 14 in, 1 out]
            n151 = Unbundle By Name(w454) -> ("Horizontal"=w450:i32, "Vertical"=w449:i32)
            n152 = Unbundle By Name(w455) -> ("button 1"=w452:bool, "button 2"=w453:bool)
            n153 = And(x=w452, y=w453) -> (x .and. y?=w451:bool)
            n154 = case shown="True" w451 {
              tunnel: w450 -> [_ w461]
              tunnel: w449 -> [_ w460]
              tunnel: w448 -> [w459 w463]
              tunnel: [w459 w462] -> w447
              frame False {
              }
              frame True {
                n155 = Bundle By Name(cluster=w463, "FP.Step.X"=w461, "FP.Step.Y"=w460) -> (w462:T5)
                n156 = local write "X"(w461) -> ()
                n157 = local write "Y"(w460) -> ()
              }
            }
          }
          frame "Assertion" {
            n158 = call-poly <vilib>:"Acquire Input Data.vi"("device ID"=w476, "error in (no error)"=w479) -> ("button info"=w475:T14, "error out"=w478:errorcluster)  [unwired: 14 in, 2 out]
            n159 = Unbundle By Name(w470) -> ("FP.Step.Left"=w468:i16, "FP.Step.Top"=w467:i16, "FP.Step.Width"=w466:i16, "FP.Step.Height"=w465:i16, "FP.Step.Control Name"=w469:string)
            n160 = Unbundle By Name(w475) -> ("button 1"=w473:bool, "button 2"=w474:bool)
            n161 = And(x=w473, y=w474) -> (x .and. y?=w472:bool)
            n162 = call "Convert to Rectangle.vi"("Height"=w465, "Width"=w466, "Top"=w467, "Left"=w468) -> ("Rectangle"=w464:T15)  [unwired: 7 in]
            n163 = case shown="True" w472 {
              tunnel: w470 -> [w480 w488]
              tunnel: [w480 w483] -> w471
              tunnel: w469 -> [_ w487]
              tunnel: w464 -> [_ w484]
              tunnel: w478 -> [w481 w491]
              tunnel: [w481 w490] -> w477
              frame False {
              }
              frame True {
                n164 = call "Get Active VI of Active Project.vi"("error in (no error)"=w491) -> ("error out"=w493:errorcluster, "Active VI Ref"=w489:refnum<vi>)  [unwired: 9 in]
                n165 = call "Get Control Ref by Name.vi"("error in (no error)"=w493, "Name"=w487, "VI Ref"=w489) -> ("error out"=w492:errorcluster, "Ctl Ref"=w486:refnum<vi>)  [unwired: 6 in, 1 out]
                n166 = call "Get Control Portion Image.vi"("error in (no error)"=w492, "subset rect"=w484, "Ctl Ref"=w486) -> ("error out"=w490:errorcluster, "Ctl Portion Picture"=→"Expected Image":picture, "Ctl Portion Image Data"=w482:T9)  [unwired: 5 in, 1 out]
                n167 = Bundle By Name(cluster=w488, "FP.Step.Expected Image"=w482) -> (w483:T5)
              }
            }
          }
          frame Default {
          }
        }
      }
      frame "---------- Macro ----------" {
        # "Do not put any code in this frame.\n(It is a separator no-op. You can make a copy of this frame to create a new Macro frame)"
        n168 = call "Enqueue Multiple States.vi"("queue in"=w496) -> ()  [unwired: 14 in, 1 out]
      }
      frame "Macro: Initialize" {
        w499 = "Data: Initialize\nInitialize Core Data\nUI: Initialize\nUI: Front Panel State >> Open"  # Data: Initialize Initialize Core Data UI: Initialize UI: Front Panel State >> Open
        # "Initialization Macro\n(This is called once, when the VI starts)"
        n169 = call "Enqueue Multiple States.vi"("State(s) at Front"=w499, "queue in"=w501) -> ()  [unwired: 13 in, 1 out]
      }
      frame "Macro: Exit" {
        # "Exit Macro\n(This is called once, when the VI exits)"
        n170 = Unbundle By Name(w511) -> ("Core.Close Panel on Exit?"=w510:bool)
        n171 = Select(t="UI: Front Panel State >> Close\n", s=w510, f="") -> (s? t:f=w506:string)
        n172 = Concatenate Strings("UI: Uninitialize\n", w506, "Data: Cleanup\nExit") -> (w504:string)
        n173 = call "Enqueue Multiple States.vi"("State(s) at Front"=w504, "queue in"=w507) -> ()  [unwired: 13 in, 1 out]
      }
    }
  }
  n174 = Merge Errors(w15, w16) -> (w14:errorcluster)
  n175 = Release Queue(queue=w12, error in (no error)=w14) -> (error out=→"error out":errorcluster)  [unwired: 1 in, 2 out]
  n176 = Unbundle By Name(w8) -> ("Step"=→"Step":refnum<class "Step.lvclass">, "OK?"=→"OK?":bool)
